vi "Test3.vi"() -> ()   [LabVIEW 2017]
panel:
  out "Output2":i32
  out "Output":i32
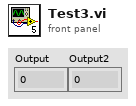
[diagram p1: front panel]
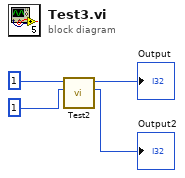
[diagram p0: block diagram]
diagram:
  n1 = call "Test2.vi"("B"=1, "A"=1) -> ("D"=→"Output2":i32, "C"=→"Output":i32)  [unwired: 8 in]
